vi "Record_Video_Example.vi"() -> ()   [LabVIEW 2022 SP3]
uses:
  Camera enum/Camera enum.ctl
  Camera enum/Camera resolution.ctl
panel:
  in  "Seconds of Video":i32
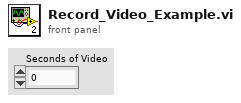
[diagram p1: front panel]
types:
  T1 = typedef "Camera enum.ctl" = string
  T2 = typedef "Camera resolution.ctl" = u8
  T3 = typedef "LVDateTimeRec.ctl" = cluster{"fractional second":dbl, "second":i32, "minute":i32, "hour":i32, "day of month":i32, "month":i32, "year":i32, "day of week":i32, "day of year":i32, "DST":i32}
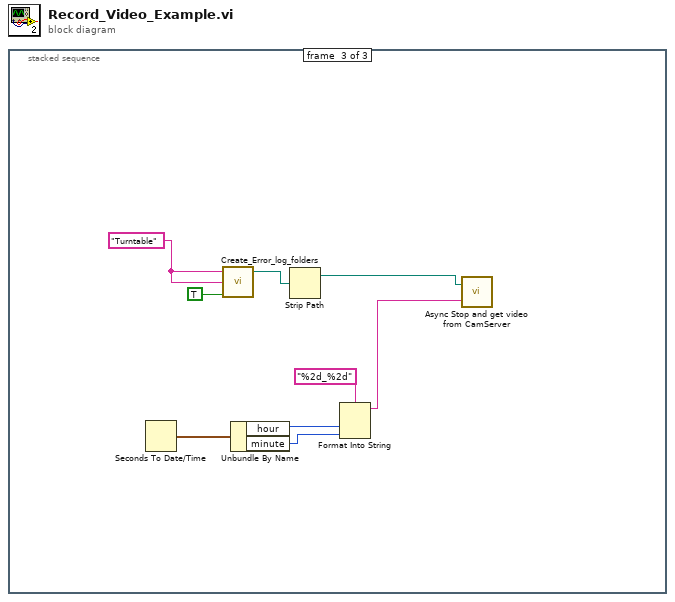
[diagram p0: block diagram]
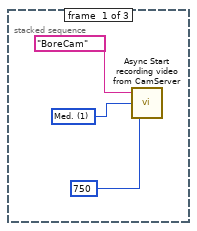
[diagram p2: hidden frame]
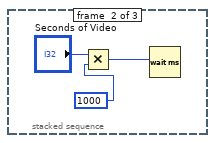
[diagram p3: hidden frame]
diagram:
  n1 = stacked-sequence {
    frame #0 {
      w2 = T2 1 items=["Low", "Med.", "High", "Max."] ("Resolution")
      n2 = call "Async Start recording video from CamServer.vi"("Quality"=750, "Resolution"=w2, "Camera"=T1 "BoreCam") -> ()  [unwired: 1 out]
    }
    frame #1 {
      n3 = Multiply(x="Seconds of Video", y=1000) -> (x*y=w5:i32)
      n4 = Wait (ms)(milliseconds to wait=w5) -> ()  [unwired: 1 out]
    }
    frame #2 {
      w8 = "Turntable" ("Input Element")
      n5 = Seconds To Date/Time() -> (date time rec=w13:T3)  [unwired: 2 in]
      n6 = call "Create_Error_log_folders.vi"("Log Filename"=w8, "Log Folder"=w8, "Per Day Log File?"=TRUE) -> ("Local Log File"=w7:path)  [unwired: 3 in, 1 out]
      n7 = Unbundle By Name(w13) -> ("hour"=w12:i32, "minute"=w11:i32)
      n8 = Strip Path(path=w7) -> (stripped path=w15:path)  [unwired: 1 out]
      n9 = Format Into String(format string="%2d_%2d", w12, w11) -> (resulting string=w14:string)  [unwired: 2 in, 1 out]
      n10 = call "Async Stop and get video from CamServer.vi"("Video name"=w14, "Video directory path"=w15) -> ()  [unwired: 1 out]
    }
  }
